vi "Pre Launch Init.vi"(11 "Stepper in":refnum<class "Stepper.lvclass">) -> (0 "error out":errorcluster, 3 "Stepper out":refnum<class "Stepper.lvclass">)   [LabVIEW 2015, in "Stepper.lvclass"]
doc: "(<B>Filename</B>: Actor Framework.lvlib:Actor.lvclass:Pre Launch Init.vi)\n\nDefines behavior that occurs after the Launch Actor method is invoked but before the actor's Actor Core method begins running.\n\nThe Pre Launch Init method is guaranteed to finish before the Launch Actor method returns to its caller and before the actor itself receives any messages. Any references that the Pre Launch Init method obtains are guaranteed to have the same lifetime as the actor itself. Any errors that the Pre Launch Init method returns will abort the launch.\n\nBy default, this method does nothing. A descendant class may override it to define behavior."
uses:
  Stepper.lvclass
  <vilib>/LabVIEW Targets/FPGA/cRIO/shared/nicrio_ModuleControls/nicrio_cRIO-9501_MicrostepRate.ctl
  <vilib>/LabVIEW Targets/FPGA/cRIO/shared/nicrio_ModuleControls/nicrio_cRIO-9501_CurrentReducPer.ctl
  Stepper.lvclass/Stepper.ctl
  CO2 Actor/CO2 Actor.lvclass
panel:
  in  "PID":cluster{"P":dbl, "I":dbl, "D":dbl}={"P"=1.0, "I"=0.5, "D"=0.5}
  in  "Current Reduction Delay":u16=100
  in  "Current Reduction Percentage":T1=enum."25 %"
  in  "Rated Phase Current":fxp<+/-,12,4>=0.3984375 format="%#_10g"
  in  "Microstepping Rate":T2
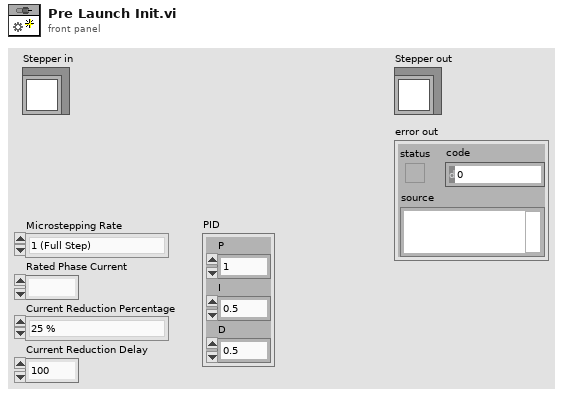
[diagram p1: front panel]
types:
  T1 = typedef "nicrio_cRIO-9501_CurrentReducPer.ctl" = enum8{"0 % (No Reduction)", "25 %", "50 %"}
  T2 = typedef "nicrio_cRIO-9501_MicrostepRate.ctl" = enum8{"1 (Full Step)", "2 (Half Step)", "4", "8", "16", "32", "64", "128", "256"}
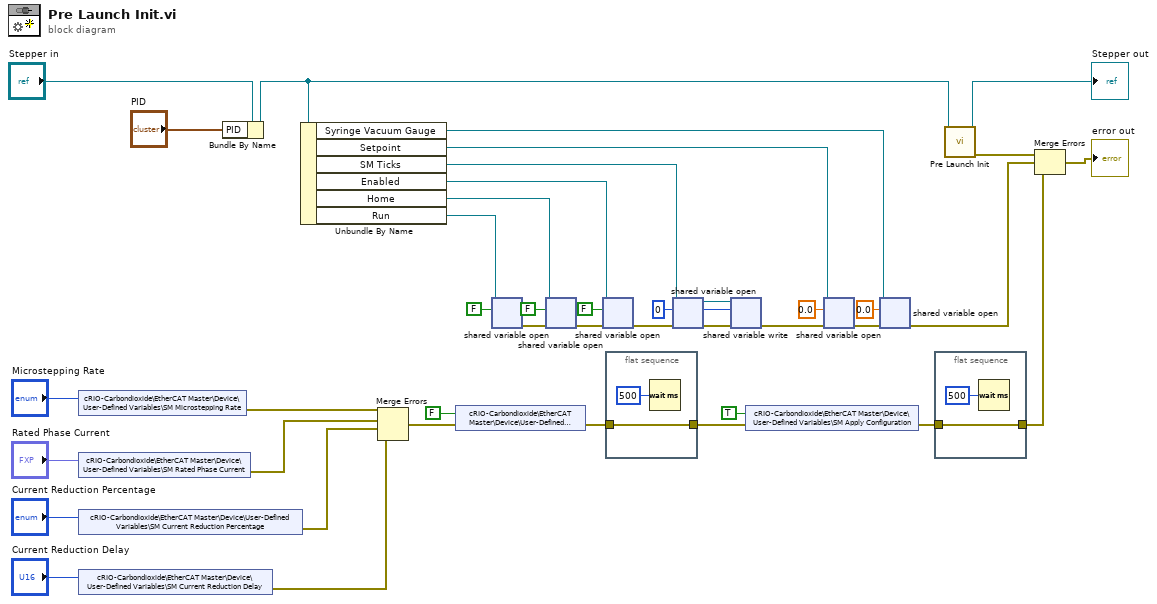
[diagram p0: block diagram]
diagram:
  w15 = i16 0
  n1 = shared-variable "cRIO-Carbondioxide\\EtherCAT Master\\Device\\User-Defined Variables\\SM Microstepping Rate"("Microstepping Rate") -> (error out=w34:errorcluster)  [unwired: 1 in]
  n2 = shared-variable "cRIO-Carbondioxide\\EtherCAT Master\\Device\\User-Defined Variables\\SM Rated Phase Current"("Rated Phase Current") -> (error out=w37:errorcluster)  [unwired: 1 in]
  n3 = shared-variable "cRIO-Carbondioxide\\EtherCAT Master\\Device\\User-Defined Variables\\SM Current Reduction Percentage"("Current Reduction Percentage") -> (error out=w35:errorcluster)  [unwired: 1 in]
  n4 = shared-variable "cRIO-Carbondioxide\\EtherCAT Master\\Device\\User-Defined Variables\\SM Current Reduction Delay"("Current Reduction Delay") -> (error out=w36:errorcluster)  [unwired: 1 in]
  n5 = Bundle By Name(cluster="Stepper in", "PID"="PID") -> (w14:refnum<class "Stepper.lvclass">)
  n6 = Unbundle By Name(w14) -> ("Syringe Vacuum Gauge"=w24:refnum<k21>, "Setpoint"=w21:refnum<k21>, "SM Ticks"=w19:refnum<k21>, "Enabled"=w13:refnum<k21>, "Home"=w8:refnum<k21>, "Run"=w5:refnum<k21>)
  n7 = Merge Errors(w34, w37, w35, w36) -> (w40:errorcluster)
  n8 = shared-variable "cRIO-Carbondioxide\\EtherCAT Master\\Device\\User-Defined Variables\\SM Enable Drive"(FALSE ("Enable Drive"), error in=w40) -> (error out=w4:errorcluster)
  n9 = shared-variable-open(w5, FALSE ("Enable Drive")) -> (w6:errorcluster)  [unwired: 2 in, 1 out]
  n10 = shared-variable-open(w8, w6, FALSE ("Enable Drive")) -> (w9:errorcluster)  [unwired: 1 in, 1 out]
  n11 = shared-variable-open(w13, w9, FALSE ("Enable Drive")) -> (w12:errorcluster)  [unwired: 1 in, 1 out]
  n12 = flat-sequence {
    tunnel: w4 -> [w43]
    tunnel: [w43] -> w3
    frame #0 {
      n13 = Wait (ms)(milliseconds to wait=u32 500) -> ()  [unwired: 1 out]
    }
  }
  n14 = shared-variable-open(w19, w12, w15) -> (w17:refnum<k21>, w18:errorcluster)  [unwired: 1 in]
  n15 = shared-variable-write(w17, w18, w15) -> (w16:errorcluster)  [unwired: 1 out]
  n16 = shared-variable "cRIO-Carbondioxide\\EtherCAT Master\\Device\\User-Defined Variables\\SM Apply Configuration"(TRUE ("Apply Configuration"), error in=w3) -> (error out=w2:errorcluster)
  n17 = shared-variable-open(w21, w16, 0.0) -> (w22:errorcluster)  [unwired: 1 in, 1 out]
  n18 = shared-variable-open(w24, w22, 0.0) -> (w25:errorcluster)  [unwired: 1 in, 1 out]
  n19 = flat-sequence {
    tunnel: w2 -> [w45]
    tunnel: [w45] -> w1
    frame #0 {
      n20 = Wait (ms)(milliseconds to wait=u32 500) -> ()  [unwired: 1 out]
    }
  }
  n21 = call-parent "Pre Launch Init.vi"("CO2 Actor in"=w14) -> ("error out"=w41:errorcluster, "CO2 Actor out"=→"Stepper out":refnum<class "Stepper.lvclass">)  [unwired: 9 in]
  n22 = Merge Errors(w41, w25, w1) -> (→"error out":errorcluster)
